vi "TurnSmooth.vi"(5 "Min Power":dbl, 6 "First Time?":bool, 7 "Target Range":dbl, 8 "Current Position":dbl, 9 "Target Position":dbl, 10 "Slow Range":dbl, 11 "Motor Power In":dbl) -> (0 "Done":bool, 3 "Motor Power Out":dbl)   [LabVIEW 2015]
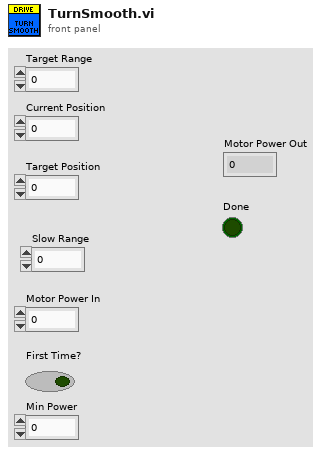
[diagram p1: front panel]
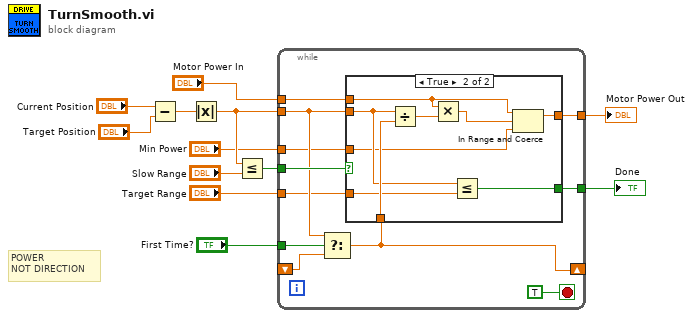
[diagram p0: block diagram]
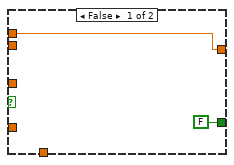
[diagram p2: hidden frame]
diagram:
  # "POWER\nNOT DIRECTION"
  n1 = Subtract(x="Current Position", y="Target Position") -> (x-y=w9:dbl)
  n2 = Absolute Value(x=w9) -> (abs(x)=w5:dbl)
  n3 = Less Or Equal?(x=w5, y="Slow Range") -> (x <= y?=w8:bool)
  n4 = while {
    tunnel: "Motor Power In" -> [w23]
    tunnel: w8 -> [w22]
    tunnel: w5 -> [w16]
    tunnel: [w21] -> w6
    tunnel: "First Time?" -> [w19]
    shift-right: [w18] -> _
    shift-left: _ -> [w17]
    tunnel: [w15] -> w3
    tunnel: "Target Range" -> [w14]
    tunnel: "Min Power" -> [w13]
    stop <- TRUE stop-if-true
    n5 = Select(t=w16, s=w19, f=w17) -> (s? t:f=w18:dbl)
    n6 = case shown="True" w22 {
      tunnel: w23 -> [w25 w31]
      tunnel: [w25 w34] -> w21
      tunnel: w16 -> [_ w29]
      tunnel: w18 -> [_ w30]
      tunnel: [FALSE w27] -> w15
      tunnel: w14 -> [_ w28]
      tunnel: w13 -> [_ w26]
      frame False {
      }
      frame True {
        n7 = Divide(x=w29, y=w30) -> (x/y=w33:dbl)
        n8 = Multiply(x=w31, y=w33) -> (x*y=w32:dbl)
        n9 = Less Or Equal?(x=w29, y=w28) -> (x <= y?=w27:bool)
        n10 = In Range and Coerce(upper limit=w31, x=w32, lower limit=w26) -> (coerced(x)=w34:dbl)  [unwired: 1 out]
      }
    }
  }
  "Motor Power Out" <- w6
  "Done" <- w3
